vi "Load - Pass - State Machine.vi"   [LabVIEW 2013]
uses:
  typedefs/singleUseSubstate.ctl
  typedefs/fg_typedef.ctl
  typedefs/subStates.ctl
types:
  T1 = typedef "singleUseSubstate.ctl" = enum16{"null", "wait", "shift high", "shift low", "extend shooter", "retract shooter", "close latch", "open latch"}
  T2 = typedef "subStates.ctl" = enum16{"null", "wait", "driver control", "auto", "manual override", "hold position", "rotate", "pickup", "pass", "load-shoot", "load-pass", "goto shoot", "shoot", "cancel", "end"}
  T3 = typedef "fg_typedef.ctl" = enum16{"Get", "Set"}
  T4 = typedef "WPI_DigitalInputDevRef.ctl" = cluster{"DevStatus":errorcluster, "DIO Channel":T5, "Digital Module":T6}
  T5 = typedef "FPGA_DIOChannel.ctl" = enum8{"DIO 1", "DIO 2", "DIO 3", "DIO 4", "DIO 5", "DIO 6", "DIO 7", "DIO 8", "DIO 9", "DIO 10", "DIO 11", "DIO 12", "DIO 13", "DIO 14", "Invalid"}
  T6 = typedef "FPGA_TypedefDigitalModule.ctl" = enum16{"Digital Module 1", "Digital Module 2"}
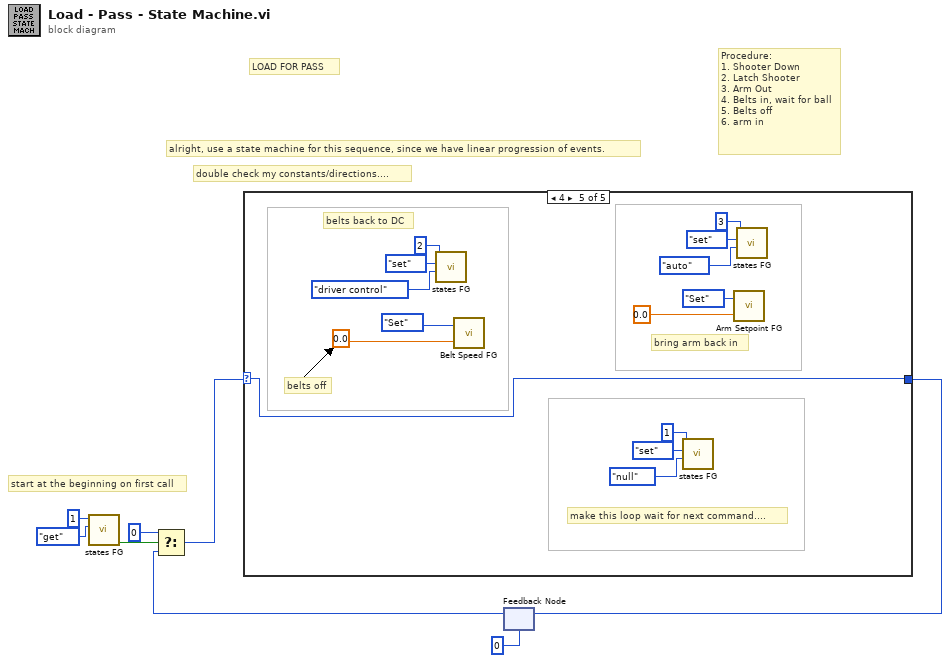
[diagram p0: block diagram]
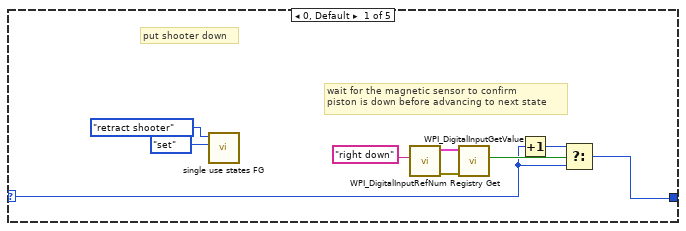
[diagram p2: hidden frame]
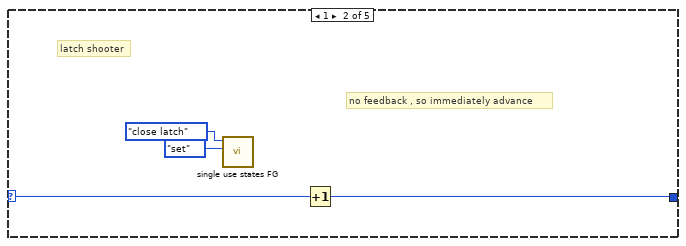
[diagram p3: hidden frame]
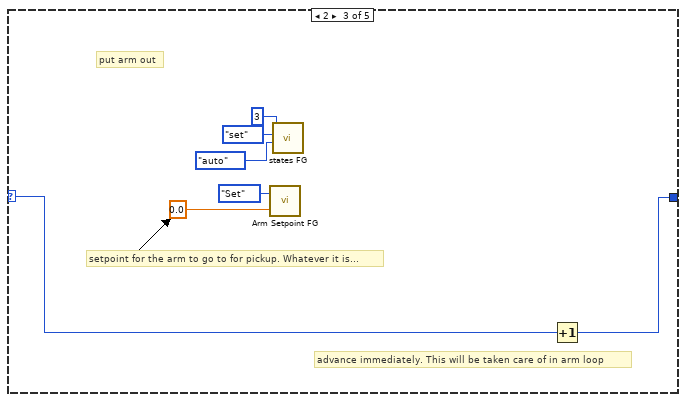
[diagram p4: hidden frame]
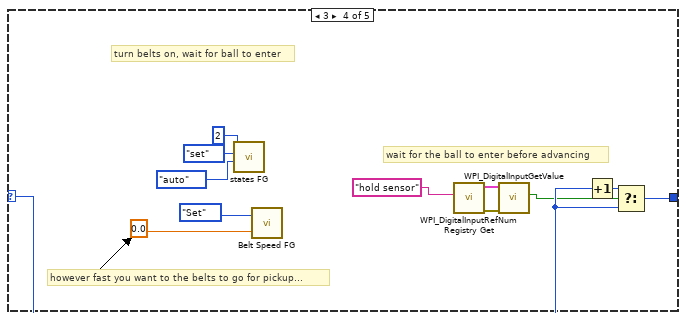
[diagram p5: hidden frame]
diagram:
  # "start at the beginning on first call"
  # "double check my constants/directions...."
  # "LOAD FOR PASS"
  # "Procedure: \n1. Shooter Down\n2. Latch Shooter\n3. Arm Out\n4. Belts in, wait for ball\n5. Belts off\n6. arm in"
  # "alright, use a state machine for this sequence, since we have linear progression of events."
  n1 = call "states FG.vi"("menu (get)"=enum16{"set", "get"}."get", "Loop ID"=1) -> ("first call?"=w1:bool)  [unwired: 6 in, 3 out]
  n2 = feedback #1(0) -> (w4:i32)
  n3 = Select(t=0, s=w1, f=w4) -> (s? t:f=w3:i32)
  n4 = case shown="4" w3 {
    selector: w3 -> [w11 w21 w23 w31 w41]
    tunnel: [w9 w18 w22 w32 w41] -> w7
    frame 0, Default {
      # "wait for the magnetic sensor to confirm \npiston is down before advancing to next state"
      # "put shooter down"
      n5 = call "single use states FG.vi"("menu (get)"=enum16{"set", "get"}."set", "substate"=singleUseSubstate."retract shooter") -> ()  [unwired: 6 in, 4 out]
      n6 = call <vilib>:"WPI_DigitalInputRefNum Registry Get.vi"("refnum name"="right down") -> ("error out"=w14:errorcluster, "DigitalInputDevRef"=w13:T4)  [unwired: 9 in]
      n7 = call <vilib>:"WPI_DigitalInputGetValue.vi"("error in (no error)"=w14, "DigitalInputDevRef"=w13) -> ("Value"=w12:bool)  [unwired: 7 in, 2 out]
      n8 = Increment(x=w11) -> (x+1=w10:i32)
      n9 = Select(t=w10, s=w12, f=w11) -> (s? t:f=w9:i32)
    }
    frame 1 {
      # "no feedback , so immediately advance"
      # "latch shooter"
      n10 = call "single use states FG.vi"("menu (get)"=enum16{"set", "get"}."set", "substate"=singleUseSubstate."close latch") -> ()  [unwired: 6 in, 4 out]
      n11 = Increment(x=w21) -> (x+1=w18:i32)
    }
    frame 2 {
      # "advance immediately. This will be taken care of in arm loop"
      # "setpoint for the arm to go to for pickup. Whatever it is..."
      # "put arm out"
      n12 = call "Arm Setpoint FG.vi"("Setpoint In"=0.0, "Menu"=fg_typedef."Set") -> ()  [unwired: 1 out]
      n13 = call "states FG.vi"("subState in"=subStates."auto", "menu (get)"=enum16{"set", "get"}."set", "Loop ID"=3) -> ()  [unwired: 5 in, 4 out]
      n14 = Increment(x=w23) -> (x+1=w22:i32)
    }
    frame 3 {
      # "wait for the ball to enter before advancing"
      # "however fast you want to the belts to go for pickup..."
      # "turn belts on, wait for ball to enter"
      n15 = call "states FG.vi"("subState in"=subStates."auto", "menu (get)"=enum16{"set", "get"}."set", "Loop ID"=2) -> ()  [unwired: 5 in, 4 out]
      n16 = call "Belt Speed FG.vi"("Speed In"=0.0 ("Setpoint In"), "Menu"=fg_typedef."Set") -> ()  [unwired: 1 out]
      n17 = call <vilib>:"WPI_DigitalInputRefNum Registry Get.vi"("refnum name"="hold sensor") -> ("error out"=w34:errorcluster, "DigitalInputDevRef"=w33:T4)  [unwired: 9 in]
      n18 = call <vilib>:"WPI_DigitalInputGetValue.vi"("error in (no error)"=w34, "DigitalInputDevRef"=w33) -> ("Value"=w29:bool)  [unwired: 7 in, 2 out]
      n19 = Increment(x=w31) -> (x+1=w30:i32)
      n20 = Select(t=w30, s=w29, f=w31) -> (s? t:f=w32:i32)
    }
    frame 4 {
      # "make this loop wait for next command...."
      # "bring arm back in"
      # "belts back to DC"
      # "belts off"
      n21 = call "states FG.vi"("subState in"=subStates."driver control", "menu (get)"=enum16{"set", "get"}."set", "Loop ID"=2) -> ()  [unwired: 5 in, 4 out]
      n22 = call "Belt Speed FG.vi"("Speed In"=0.0 ("Setpoint In"), "Menu"=fg_typedef."Set") -> ()  [unwired: 1 out]
      n23 = call "states FG.vi"("subState in"=subStates."null", "menu (get)"=enum16{"set", "get"}."set", "Loop ID"=1) -> ()  [unwired: 5 in, 4 out]
      n24 = call "Arm Setpoint FG.vi"("Setpoint In"=0.0, "Menu"=fg_typedef."Set") -> ()  [unwired: 1 out]
      n25 = call "states FG.vi"("subState in"=subStates."auto", "menu (get)"=enum16{"set", "get"}."set", "Loop ID"=3) -> ()  [unwired: 5 in, 4 out]
    }
  }
  n26 = feedback-in #1(w7) -> ()
